vi "Relink.vi"(0 "Subroutine in":refnum<class "Subroutine.lvclass">, 1 "Linked List Ref":refnum<data-value>, 2 "File Path":path, 5 "Flattened Test Executive":string, 7 "Return":string, 9 "Linked List ID":string, 11 "error in (no error)":errorcluster, 12 "Persistence in":refnum<class "IPersist.lvclass">, 13 "Compatibility Helper":refnum<class "ICompatibility Helper.lvclass">, 14 "Path Builder":refnum<class "IPath Builder.lvclass">) -> (3 "Linked List Ref out":refnum<data-value>, 6 "Flattened Test Executive out":string, 8 "Return out":string, 15 "error out":errorcluster)   [LabVIEW 2019, in "Test Executive.lvlib" / "Subroutine.lvclass"]
uses:
  <vilib>/gpm_packages/@cs/test-executive/Source/Test Executive/Subroutine/Subroutine.lvclass
  <vilib>/gpm_packages/@cs/persistence/source/IPersist/IPersist.lvclass
  <vilib>/gpm_packages/@cs/linked-list/Source/Linked List/ILinkedList/ILinked List.lvclass
  <vilib>/gpm_packages/@cs/test-executive/Source/Path Builder/IPath Builder/IPath Builder.lvclass
  <vilib>/gpm_packages/@cs/test-executive/Source/Compatibility Helper/ICompatibility Helper.lvclass
  <vilib>/gpm_packages/@cs/test-executive/Source/Test Executive/Executioner/Executioner.lvclass
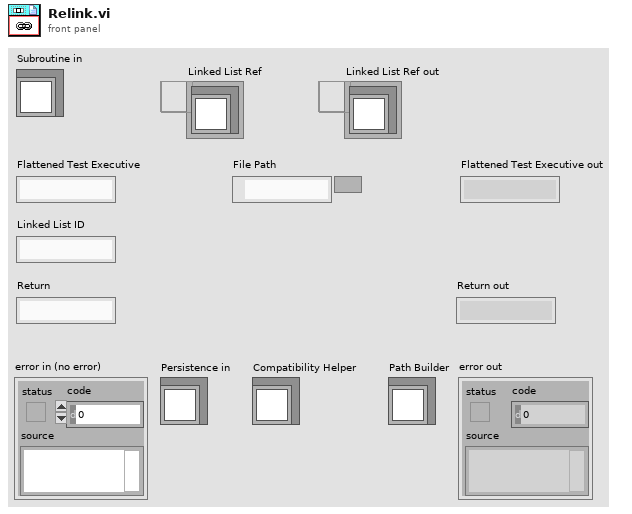
[diagram p1: front panel]
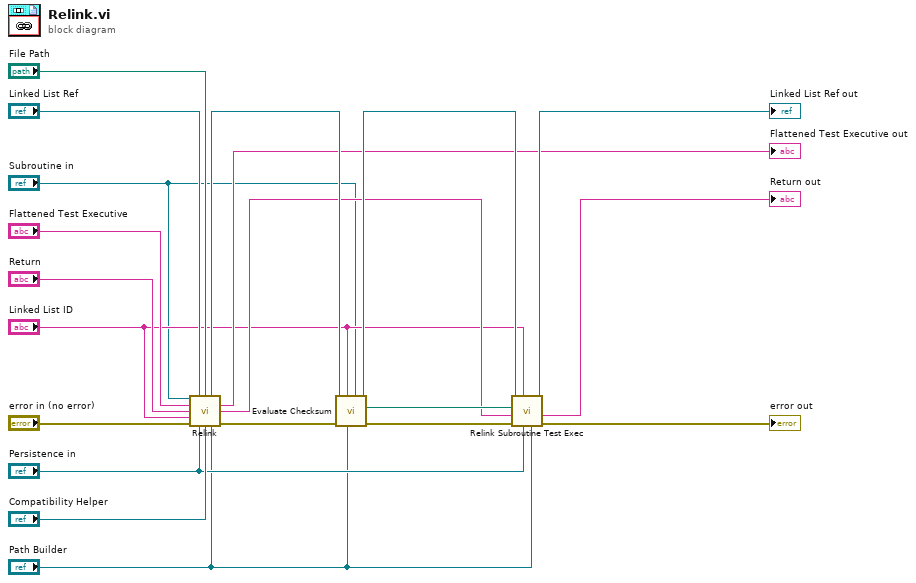
[diagram p0: block diagram]
diagram:
  n1 = call-parent "Relink.vi"("Executioner in"="Subroutine in", "Linked List Ref"="Linked List Ref", "File Path"="File Path", "Flattened Test Executive"="Flattened Test Executive", "Return"="Return", "Linked List ID"="Linked List ID", "error in (no error)"="error in (no error)", "Persistence in"="Persistence in", "Compatibility Helper"="Compatibility Helper", "Path Builder"="Path Builder") -> ("Linked List Ref out"=w13:refnum<data-value>, "Flattened Test Executive out"=→"Flattened Test Executive out":string, "Return out"=w7:string, "error out"=w14:errorcluster)  [unwired: 2 in]
  n2 = call <vilib>:"Evaluate Checksum.vi"("Subroutine in"="Subroutine in", "Path Builder"="Path Builder", "Linked List ID"="Linked List ID", "error in (no error)"=w14, "Linked List Ref"=w13) -> ("error out"=w12:errorcluster, "Path"=w8:path, "Linked List Ref out"=w10:refnum<data-value>)  [unwired: 3 in, 1 out]
  n3 = call <vilib>:"Relink Subroutine Test Exec.vi"("Path Builder"="Path Builder", "Persistence in"="Persistence in", "Linked List ID"="Linked List ID", "error in (no error)"=w12, "Return"=w7, "Subroutine Path"=w8, "Linked List Ref"=w10) -> ("error out"=→"error out":errorcluster, "Return out"=→"Return out":string, "Linked List Ref out"=→"Linked List Ref out":refnum<data-value>)  [unwired: 2 in]
